vi "Page_Source_Settings_Update_Display.vi"(6 "AB_Build in":refnum<class "AB_Build.lvclass">, 8 "error in (no error)":errorcluster, 9 "ctlReferences":T3, 10 "supportedFunctions":T2, 11 "AB_Source_PackedItem in":refnum<class "AB_Source_PackedItem.lvclass">) -> (0 "error out":errorcluster, 2 "parentApplies":T1, 3 "AB_Source_PackedItem out":refnum<class "AB_Source_PackedItem.lvclass">)   [LabVIEW 2020, in "AB_Source_PackedItem.lvclass"]
uses:
  <vilib>/AppBuilder/AB_Classes/Source/PackedItem/AB_Source_PackedItem.lvclass
  <resource>/Framework/Providers/Builds/AppBuilder/AB_UI_Page_Source_Settings_References.ctl
  <resource>/Framework/Providers/Builds/AppBuilder/AB_UI_Page_Source_Settings_supportedFunctions.ctl
  <vilib>/AppBuilder/AB_Parent_Applies.ctl
  <vilib>/AppBuilder/AB_Classes/Build/AB_Build.lvclass
  <vilib>/AppBuilder/AB_Classes/Source/AB_Source.lvclass
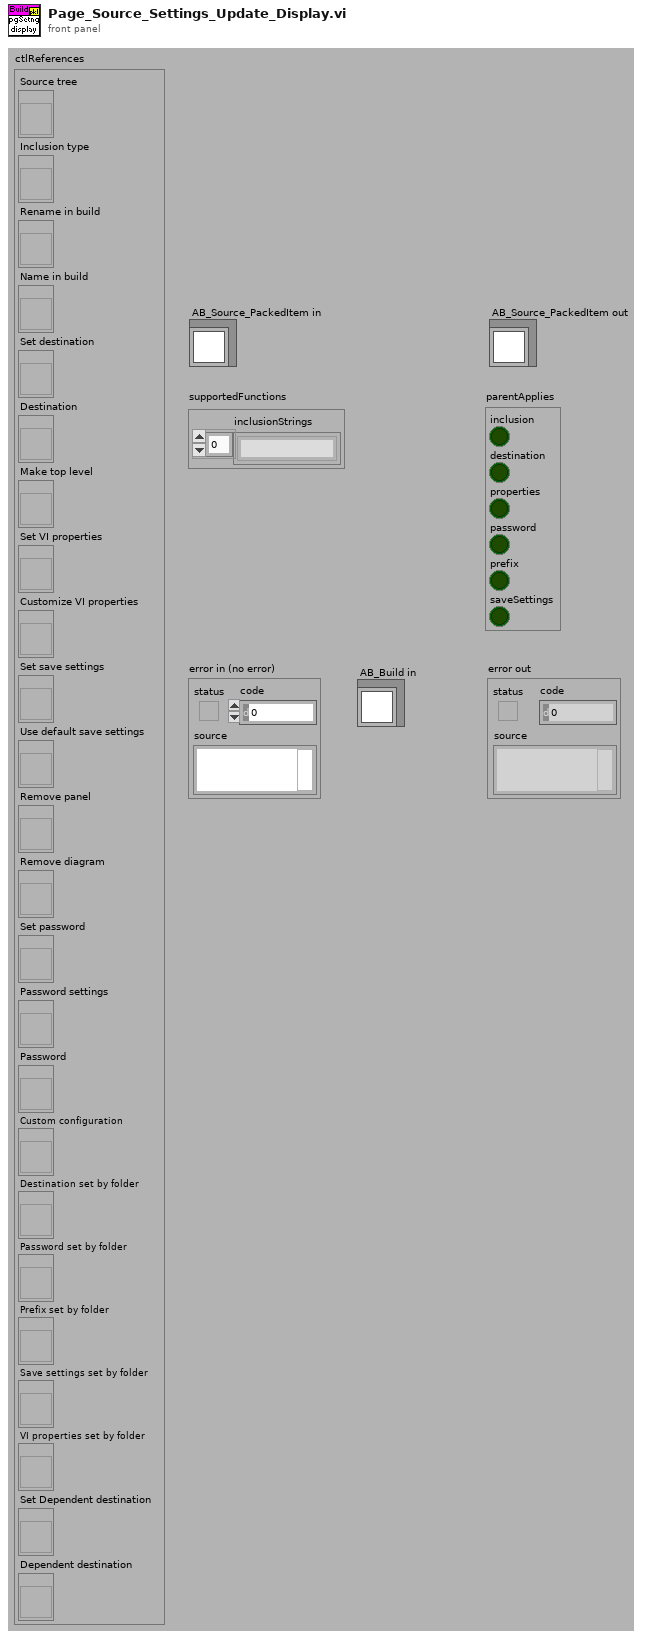
[diagram p1: front panel]
types:
  T1 = typedef "AB_Parent_Applies.ctl" = cluster{"inclusion":bool, "destination":bool, "properties":bool, "password":bool, "prefix":bool, "saveSettings":bool}
  T2 = typedef "AB_UI_Page_Source_Settings_supportedFunctions.ctl" = cluster{"inclusionStrings":string[]}
  T3 = typedef "AB_UI_Page_Source_Settings_References.ctl" = cluster{"Source tree":refnum<vi>, "Inclusion type":refnum<vi>, "Rename in build":refnum<vi>, "Name in build":refnum<vi>, "Set destination":refnum<vi>, "Destination":refnum<vi>, "Make top level":refnum<vi>, "Set VI properties":refnum<vi>, "Customize VI properties":refnum<vi>, "Set save settings":refnum<vi>, "Use default save settings":refnum<vi>, "Remove panel":refnum<vi>, "Remove diagram":refnum<vi>, "Set password":refnum<vi>, "Password settings":refnum<vi>, "Password":refnum<vi>, "Custom configuration":refnum<vi>, "Destination set by folder":refnum<vi>, "Password set by folder":refnum<vi>, "Prefix set by folder":refnum<vi>, "Save settings set by folder":refnum<vi>, "VI properties set by folder":refnum<vi>, "Set Dependent destination":refnum<vi>, "Dependent destination":refnum<vi>}
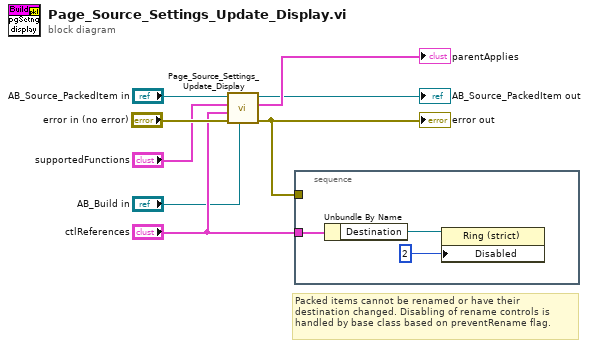
[diagram p0: block diagram]
diagram:
  # "Packed items cannot be renamed or have their destination changed. Disabling of rename controls is handled by base class based on preventRename flag."
  n1 = call-parent "Page_Source_Settings_Update_Display.vi"("AB_Build in"="AB_Build in", "error in (no error)"="error in (no error)", "ctlReferences"="ctlReferences", "supportedFunctions"="supportedFunctions", "AB_Source in"="AB_Source_PackedItem in") -> ("error out"=w2:errorcluster, "parentApplies"=→"parentApplies":T1, "AB_Source out"=→"AB_Source_PackedItem out":refnum<class "AB_Source_PackedItem.lvclass">)  [unwired: 4 in]
  "error out" <- w2
  n2 = stacked-sequence {
    tunnel: "ctlReferences" -> [w9]
    tunnel: w2 -> [_]
    frame #0 {
      n3 = Unbundle By Name(w9) -> ("Destination"=w11:refnum<vi>)
      n4 = property class="Ring (strict)"(reference=w11, "Disabled"=u8 2) -> ()  [unwired: 1 in, 2 out]
    }
  }
